vi "mlink_scan_trigger_dio_pattern.vi"(7 "trigger type":T1, 8 "error in (no error)":errorcluster, 9 "len":u8, 10 "pattern":string, 11 "connection ID":i32=-1) -> (0 "error out":errorcluster, 3 "connection ID out":i32)   [LabVIEW 2009, in "MicroDAQ.lvlib" / "mlink.lvlib"]
doc: "This function configures DIO pattern trigger for AO/AI scan operation. The function shall be called after scan initialization function. The trigger argument determines if function affects\nAO or AI trigger settings. The pattern argument must contains eight characters string with 'x', '1' or '0' defining desired DIO1...8 state. The 'x' character indicates that DIO is state is\nignored, while 0 and 1 indicated low and high state respectively. DIO pattern defines DIO\nstate in the following order DIO1, DIO2, DIO3, DIO4, DIO5, DIO6, DIO7, DIO8 e.g. pattern '11xxxxxx' is related to DIO1 and DIO2 state. If defined pattern is present on DIO1…8 AO or AI scan will start.\nThe len argument shall contain pattern string length. Value different then 8 will cause an error."
uses:
  <instrlib>/MicroDAQ/Mlink library wraper/mlink.lvlib
  <instrlib>/MicroDAQ/Tools/Trigger type.ctl
  <instrlib>/MicroDAQ/MLink32.dll
  <instrlib>/MicroDAQ/MicroDAQ.lvlib
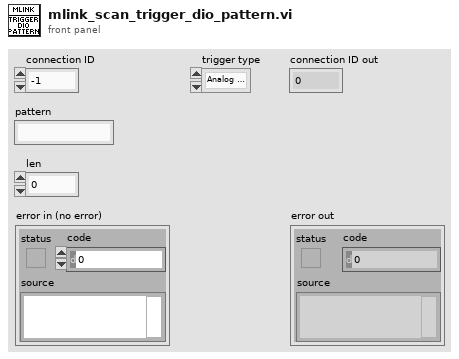
[diagram p1: front panel]
types:
  T1 = typedef "MicroDAQ.lvlib/Trigger type.ctl" = enum8{"Analog output", "Analog input"}
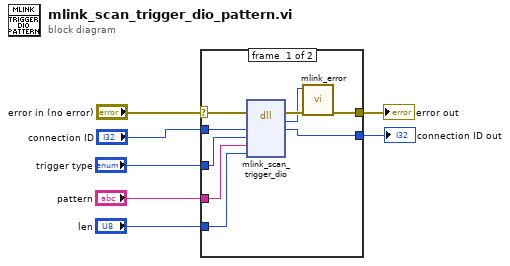
[diagram p0: block diagram]
diagram:
  n1 = case shown="No Error" "error in (no error)" {
    selector: "error in (no error)" -> [w16 w18]
    tunnel: "connection ID" -> [w15 w17]
    tunnel: [w14 w17] -> w5
    tunnel: [w11 w18] -> w4
    tunnel: "trigger type" -> [w10 _]
    tunnel: "len" -> [w9 _]
    tunnel: "pattern" -> [w8 _]
    frame #0 {
      n2 = dll-call lib="C:/Program Files (x86)/National Instruments/LabVIEW 2009/instr.lib/MicroDAQ/MLink32.dll" fn="mlink_scan_trigger_dio" ("MLink64.dll:mlink_dsp_run")(error in=w16, "link_fd"=w15, "trigger"=w10, "pattern"=w8, "len"=w9) -> (error out=w13:errorcluster, "return type"=w12:i32, "link_fd"=w14:i32)  [unwired: 5 in, 1 out]
      n3 = call <instrlib>:"mlink_error.vi"("error in (no error)"=w13, "error code"=w12) -> ("error out"=w11:errorcluster)  [unwired: 9 in]
    }
    frame #1 {
    }
  }
  "connection ID out" <- w5
  "error out" <- w4
